vi "FTW-Endpoint-Multipart-Reply.vi"(0 "FTW Endpoint":refnum<class "FTW-Endpoint.lvclass">, 5 "Multipart Message":string[](array[string]), 7 "Timeout":i32 format="%dmsec", 11 "error in":errorcluster) -> (4 "FTW Endpoint out":refnum<class "FTW-Endpoint.lvclass">, 6 "Timed out?":bool, 15 "error out":errorcluster)   [LabVIEW 2012, in "FTW-Actor.lvlib" / "FTW-Endpoint.lvclass"]
uses:
  FTW-Endpoint.lvclass
panel:
  # "Inputs"
  # "Outputs"
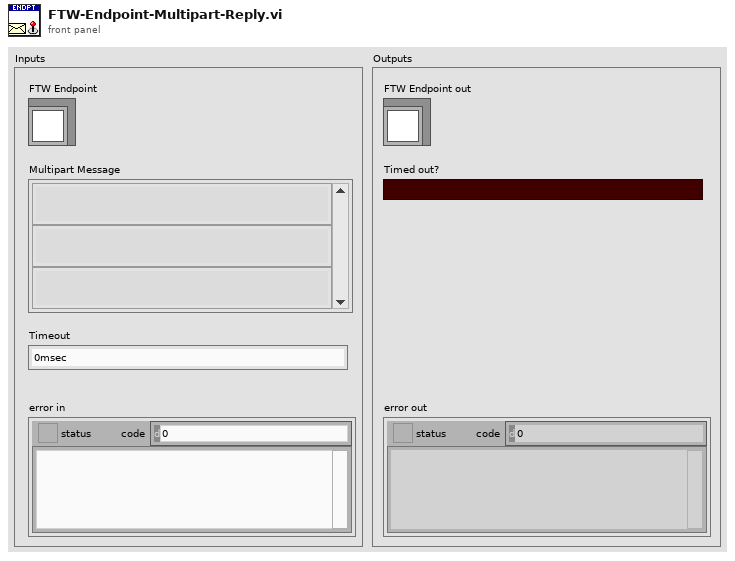
[diagram p1: front panel]
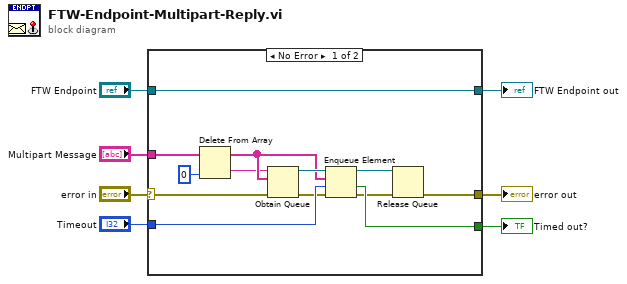
[diagram p0: block diagram]
diagram:
  n1 = case shown="No Error" "error in" {
    selector: "error in" -> [w17 w22]
    tunnel: [w8 w22] -> w7
    tunnel: [w18 w21] -> w5
    tunnel: "FTW Endpoint" -> [w18 w21]
    tunnel: "Multipart Message" -> [w14 _]
    tunnel: [w20 _] -> w2
    tunnel: "Timeout" -> [w19 _]
    frame No Error {
      n2 = Delete From Array(array=w14, index=0) -> (deleted portion=w11:string, array with subset deleted=w13:string[])  [unwired: 1 in]
      n3 = Obtain Queue(name (unnamed)=w11, element data type=w13, error in (no error)=w17) -> (queue out=w15:refnum<queue>, error out=w16:errorcluster)  [unwired: 2 in, 1 out]
      n4 = Enqueue Element(queue=w15, element=w13, timeout in ms (-1)=w19, error in (no error)=w16) -> (queue out=w10:refnum<queue>, timed out?=w20:bool, error out=w9:errorcluster)
      n5 = Release Queue(queue=w10, error in (no error)=w9) -> (error out=w8:errorcluster)  [unwired: 1 in, 2 out]
    }
    frame Error {
    }
  }
  "error out" <- w7
  "FTW Endpoint out" <- w5
  "Timed out?" <- w2
